vi "Main.vi"() -> ()   [LabVIEW 2020]
uses:
  <userlib>/_NEVSTOP/Communicable State Machine(CSM)/AdvanceAPI/CSM - Revert Arguments-Safe String.vi
  <userlib>/_NEVSTOP/Communicable State Machine(CSM)/_Support/Common/Trim Single line Text.vi
  <userlib>/_NEVSTOP/Communicable State Machine(CSM)/AdvanceAPI/CSM - Make String Arguments Safe.vi
  <userlib>/_NEVSTOP/Communicable State Machine(CSM)/AdvanceAPI/CSM - Break Down Multiple States String.vi
  <userlib>/_NEVSTOP/Communicable State Machine(CSM)/AdvanceAPI/CSM - Compact Multiple States.vi
  <userlib>/_NEVSTOP/Communicable State Machine(CSM)/AdvanceAPI/CSM - Keywords.vi
  <userlib>/_NEVSTOP/Communicable State Machine(CSM)/_Support/CSMQ/_CSMOFGV.vi
  <userlib>/_NEVSTOP/Communicable State Machine(CSM)/Communicable State Machine.lvlib
panel:
  out "State History":string
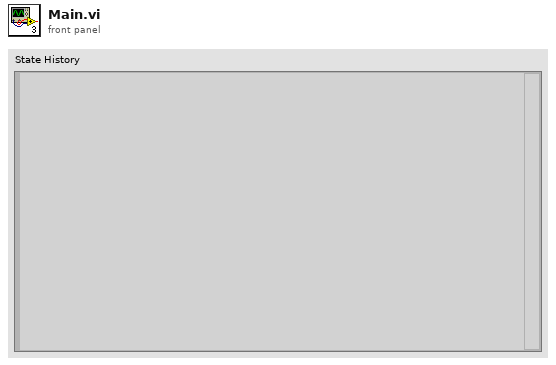
[diagram p1: front panel]
types:
  T1 = enum32{"Invalid", "Standard", "Closed", "Hidden", "Minimized", "Maximized"}
  T2 = enum32{"invalid app kind", "Development System", "Run Time System", "Student Edition", "Embedded LabVIEW", "Evaluation", "Custom"}
  T3 = typedef "Communicable State Machine.lvlib/_CSM_Response Source Message.ctl" = cluster{"‘State":string, "’Arguments":string, "’Error":errorcluster}
  T4 = cluster{"Current VI Reference":refnum<vi>, "Close Panel on Exit?":bool}
  T5 = cluster{"Core":cluster{"Current VI Reference":refnum<vi>, "Close Panel on Exit?":bool}, "Your Boolean data":bool, "Your string data":string}
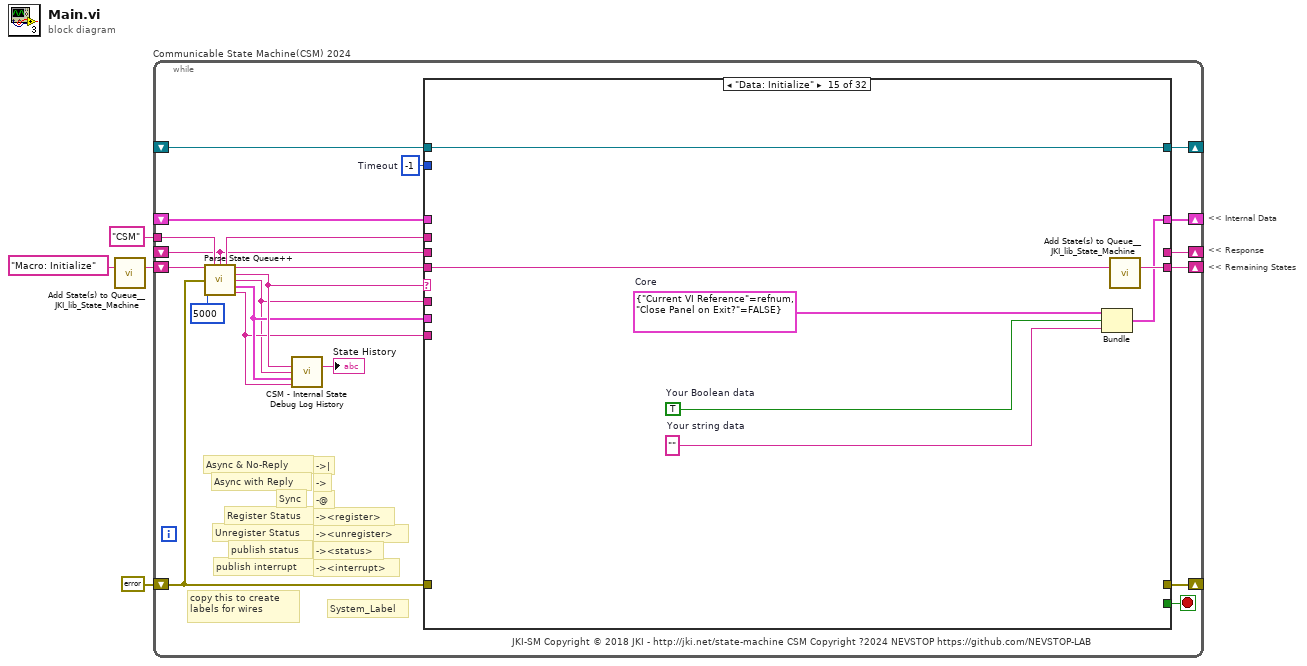
[diagram p0: block diagram]
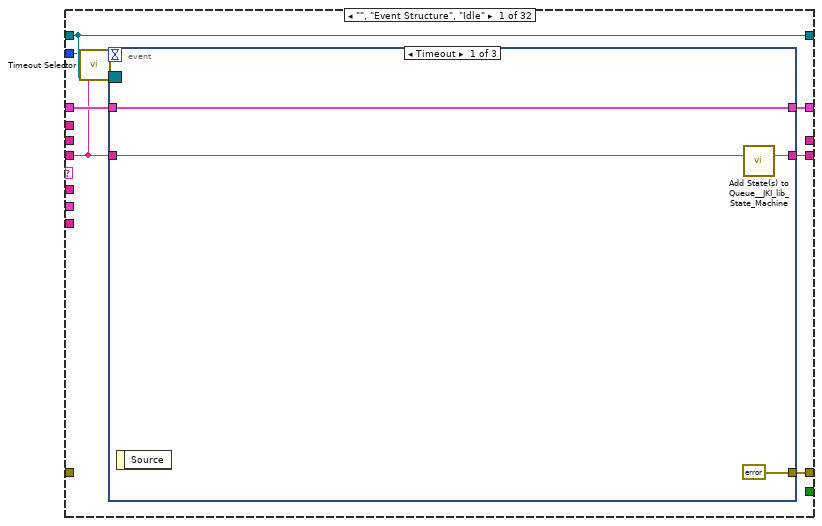
[diagram p2: hidden frame]
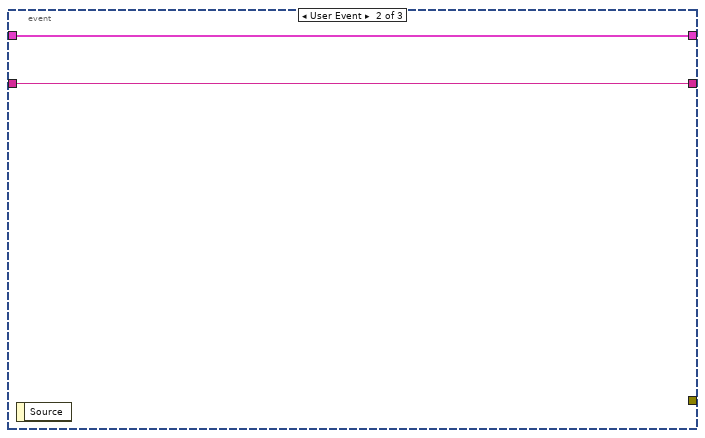
[diagram p3: hidden frame]
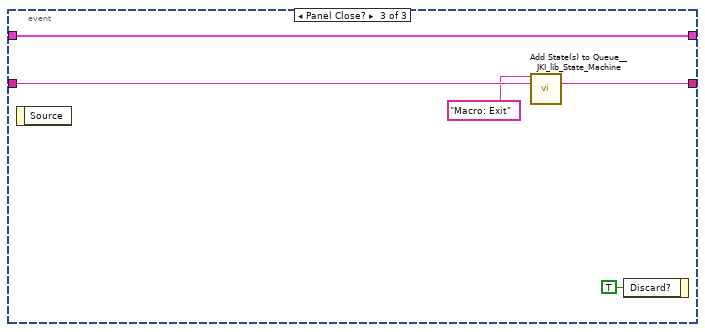
[diagram p4: hidden frame]
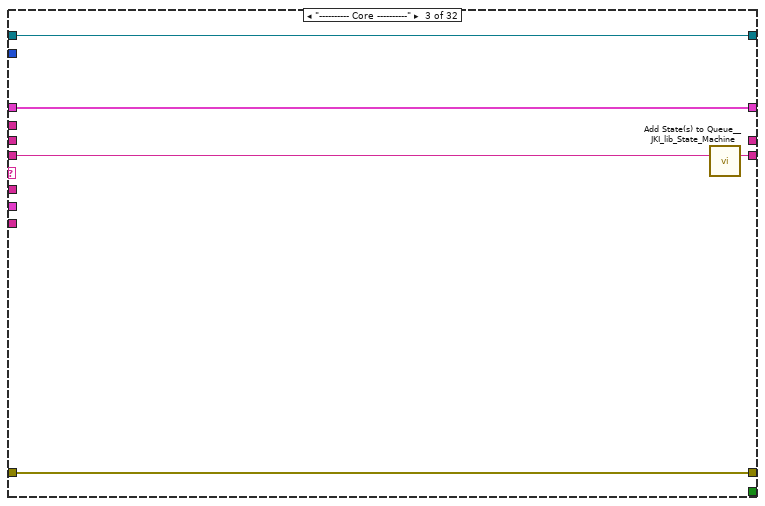
[diagram p6: hidden frame]
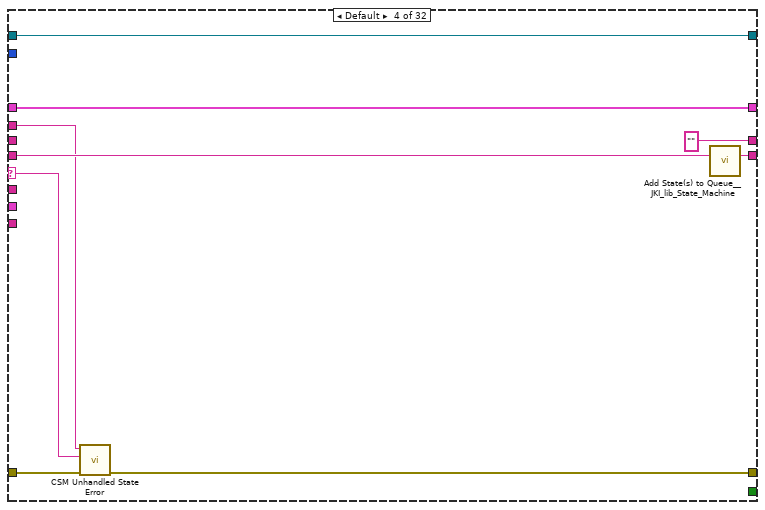
[diagram p7: hidden frame]
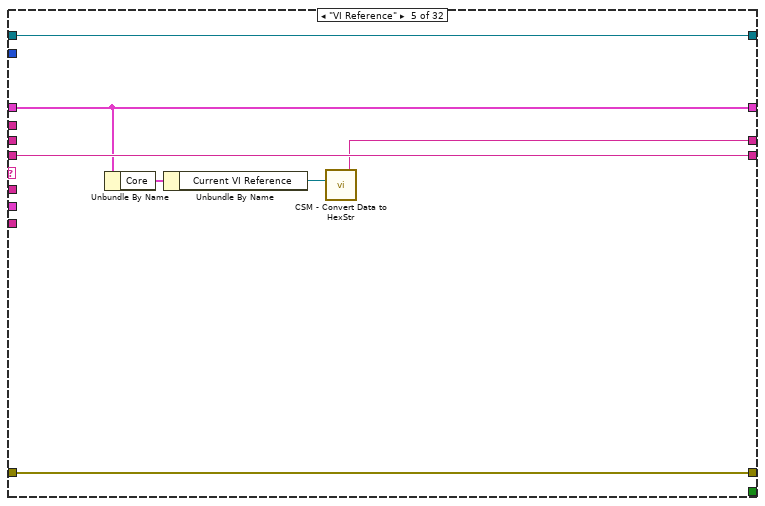
[diagram p8: hidden frame]
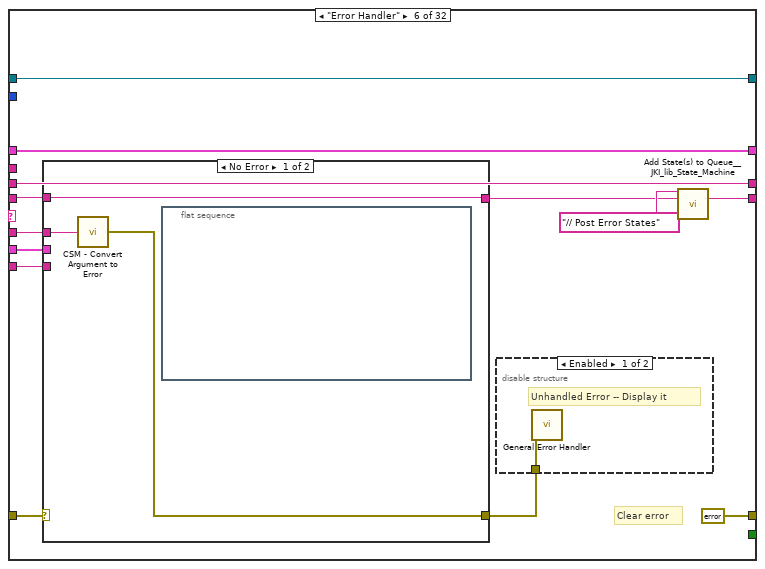
[diagram p9: hidden frame]
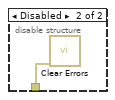
[diagram p10: hidden frame]
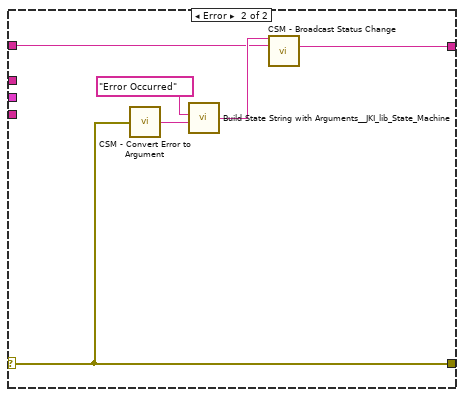
[diagram p11: hidden frame]
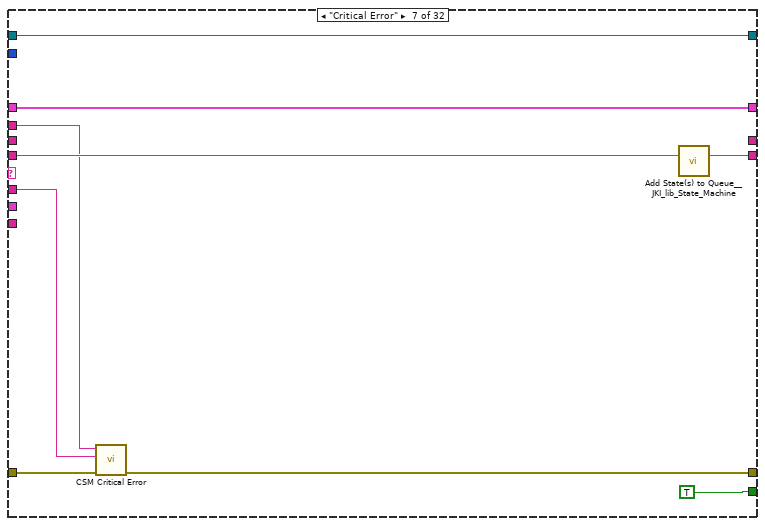
[diagram p12: hidden frame]
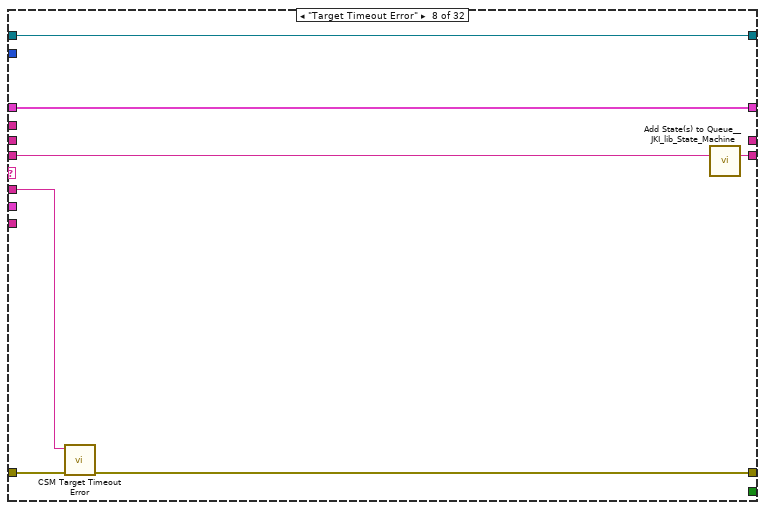
[diagram p13: hidden frame]
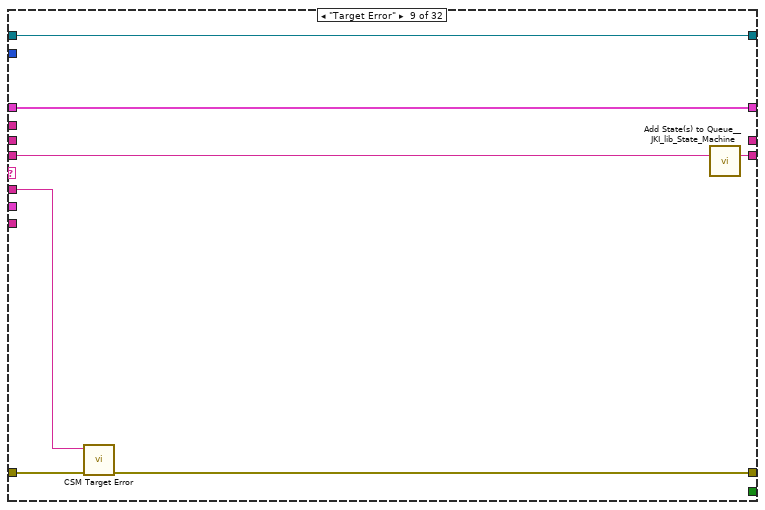
[diagram p14: hidden frame]
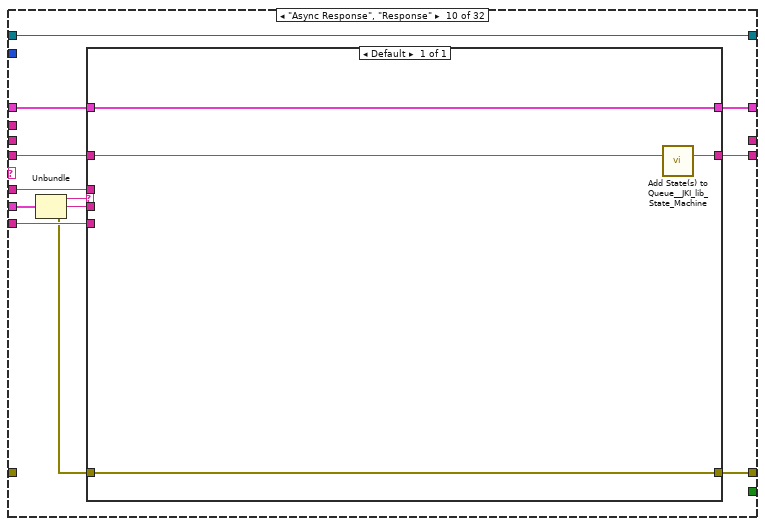
[diagram p15: hidden frame]
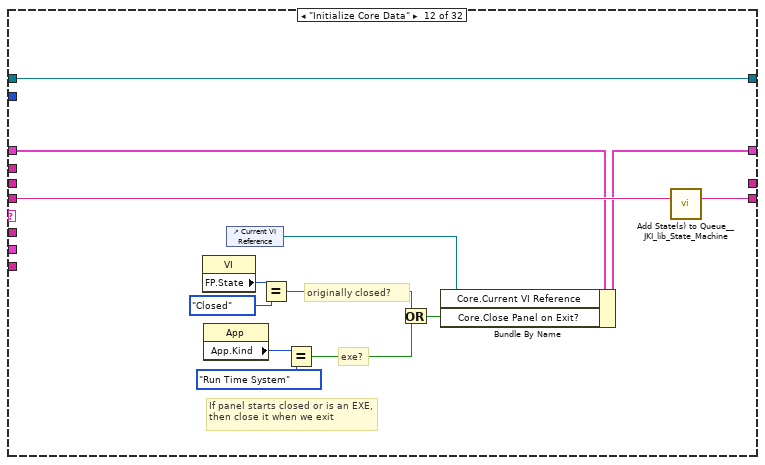
[diagram p17: hidden frame]
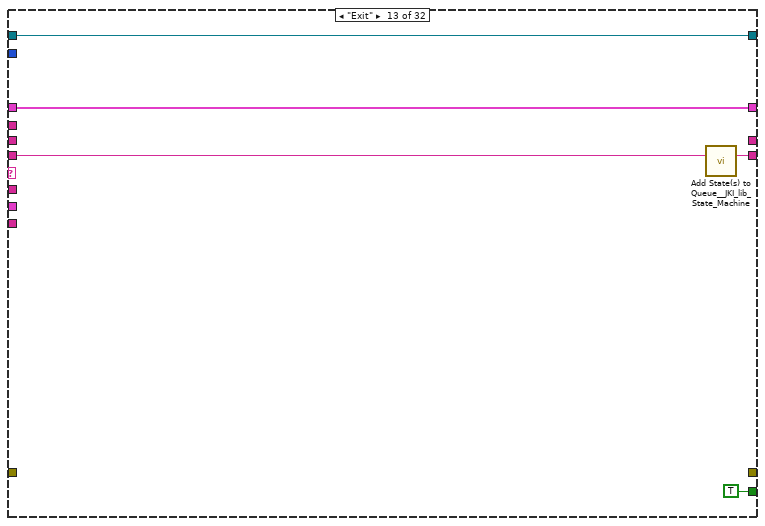
[diagram p18: hidden frame]
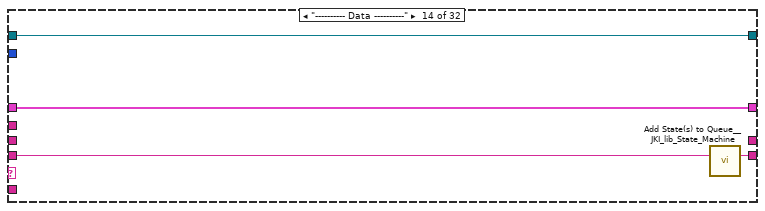
[diagram p19: hidden frame]
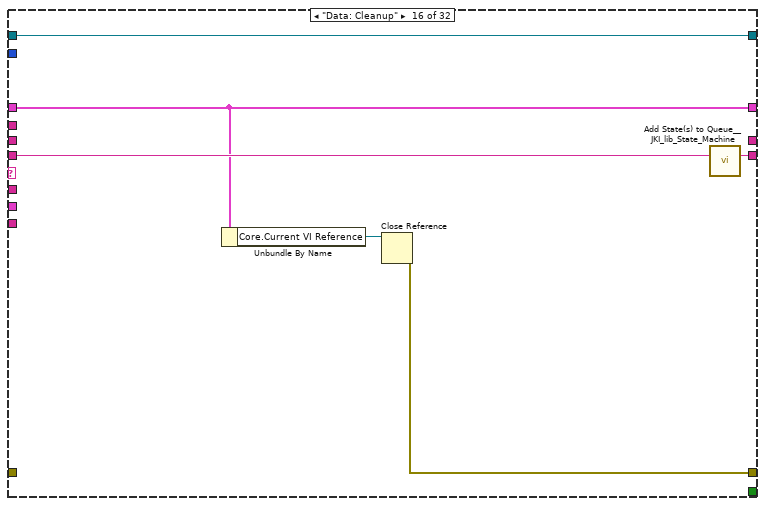
[diagram p20: hidden frame]
diagram:
  # "<< Internal Data"
  # "<< Response"
  # "<< Remaining States"
  n1 = call <vilib>:"Add State(s) to Queue__JKI_lib_State_Machine.vi"("State(s) in (\"\")"="Macro: Initialize" ("Init State(\"Macro: Initialize\")")) -> ("States Out"=w1:string)  [unwired: 14 in]
  n2 = while "Communicable State Machine(CSM) 2024" {
    shift-right: [w20] -> _
    shift-left: _ -> [w19]
    shift-right: [w23] -> _
    shift-left: errorcluster {"status"=FALSE, "code"=0, "source"=""} ("error out") -> [w17]
    shift-right: [w22] -> _
    shift-left: w1 -> [w24]
    tunnel: "CSM" ("Name(\"\" to use uuid)") -> [w12]
    shift-right: [w15] -> _
    shift-left: _ -> [w7]
    shift-right: [w14] -> _
    shift-left: _ -> [w13]
    stop <- w21 stop-if-true
    w18 = -1  # Timeout
    # "-><interrupt>"
    # "-><status>"
    # "-><unregister>"
    # "-><register>"
    # "-@"
    # "->"
    # "->|"
    # "publish interrupt"
    # "publish status"
    # "Unregister Status"
    # "Register Status"
    # "Sync"
    # "Async with Reply"
    # "Async & No-Reply"
    # "copy this to create labels for wires"
    # "System_Label"
    # "JKI-SM Copyright © 2018 JKI - http://jki.net/state-machine CSM Copyright ?2024 NEVSTOP https://github.com/NEVSTOP-LAB"
    n3 = call <userlib>:"Parse State Queue++.vi"("State Queue"=w24, "Name(\"\" to use uuid)"=w12, "Response Arguments"=w7, "Previous Error"=w17, "Response Timeout(5000ms)"=5000 ("Response Timeout(1000ms)")) -> ("Name Used"=w8:string, "Remaining States"=w25:string, "Current State"=w11:string, "Arguments"=w6:string, ">> Response Source Message >>"=w10:T3, ">> Source CSM >>"=w9:string)  [unwired: 5 in]
    n4 = call <userlib>:"CSM - Internal State Debug Log History.vi"("State"=w11, "Arguments (\"\")"=w6, ">> Response Source Message >>"=w10, "Source (\"\")"=w9) -> ("Debug Log"=→"State History":string)  [unwired: 11 in]
    n5 = case shown="\"Data: Initialize\"" w11 {
      selector: w11 -> [_ _ _ w55 _ _ _ _ _ _ _ _ _ _ _ _ _ _ _ _ _ _ _ _ _ _ _ _ _ _ _ _]
      tunnel: w25 -> [w26 w47 w52 w61 w67 w74 w100 w108 w115 w125 w134 w147 w152 w156 w163 w169 w173 w180 w184 w188 w192 w198 w209 w273 w278 w289 w292 w296 w299 w303 w307 w311]
      tunnel: w6 -> [_ _ _ _ _ w72 w96 w103 w111 w119 _ _ _ _ _ _ _ _ _ _ _ w194 w204 _ _ _ _ _ _ _ _ _]
      tunnel: w19 -> [w32 w46 w49 w59 w66 w80 w101 w106 w113 w123 w133 w141 w150 w154 _ w165 w171 w179 w183 w186 w190 w196 w206 w271 w276 w287 w291 w295 w298 w301 w305 w309]
      tunnel: [w31 _ w50 w53 w68 errorcluster {"status"=FALSE, "code"=0, "source"=""} ("error out") w93 w102 w109 w122 _ _ _ _ _ w166 _ w174 w182 _ _ w195 w207 _ _ _ _ _ _ _ _ _] -> w23
      tunnel: w17 -> [_ _ w50 w54 w68 w78 w94 w104 w110 _ _ _ _ _ _ _ _ _ _ _ _ _ _ _ _ _ _ _ _ _ _ _]
      tunnel: [w33 w47 w51 w60 w67 w76 w99 w107 w114 w126 w134 w146 w151 w155 w162 w168 w172 w180 w184 w187 w191 w197 w208 w272 w277 w288 w292 w296 w299 w302 w306 w310] -> w22
      tunnel: [_ _ _ _ _ _ TRUE _ _ _ _ _ TRUE _ _ _ _ _ _ _ _ _ _ _ _ _ _ _ _ _ _ _] -> w21
      tunnel: [w30 w46 w49 w59 w66 w80 w101 w106 w113 w124 w133 w145 w150 w154 w161 w165 w171 w179 w183 w186 w190 w196 w206 w271 w276 w287 w291 w295 w298 w301 w305 w309] -> w20
      tunnel: w18 -> [w28 _ _ _ _ _ _ _ _ _ _ _ _ _ _ _ _ _ _ _ _ _ _ _ _ _ _ _ _ _ _ _]
      tunnel: w9 -> [_ _ _ _ _ w71 _ _ _ w120 _ _ _ _ _ _ _ _ _ _ _ _ _ _ _ _ _ _ _ _ _ _]
      tunnel: w10 -> [_ _ _ _ _ w70 _ _ _ w121 _ _ _ _ _ _ _ _ _ _ _ _ _ _ _ _ _ _ _ _ _ _]
      tunnel: [_ _ _ "" w62 w69 _ _ _ _ _ _ _ _ _ _ _ _ _ _ _ _ _ _ _ _ _ "API1 Response" _ _ _ _] -> w15
      tunnel: [w29 w45 w48 w57 w65 w79 w97 w105 w112 w127 w132 w135 w148 w153 w157 w164 w170 w178 w181 w185 w189 w193 w203 w270 w274 w280 w290 w294 w297 w300 w304 w308] -> w14
      tunnel: w13 -> [w29 w45 w48 w57 w65 w79 w97 w105 w112 w127 w132 w135 w148 w153 w157 w164 w170 _ w181 w185 w189 w193 w203 w270 w274 w280 w290 w294 w297 w300 w304 w308]
      tunnel: w8 -> [_ _ _ w56 _ _ w95 _ _ _ _ _ _ _ _ _ _ w177 _ _ _ _ _ _ _ _ _ _ _ _ _ _]
      tunnel: w7 -> [_ _ _ _ _ w69 _ _ _ _ _ _ _ _ _ _ _ _ _ _ _ _ _ _ _ _ _ _ _ _ _ _]
      frame "", "Event Structure", "Idle" {
        n6 = call <userlib>:"Timeout Selector.vi"("Remaining States"=w26, "Timeout Expected"=w28) -> ("Timeout"=w27:i32)  [unwired: 5 in]
        n7 = event shown="[0] Timeout" {
          selector: w29 -> [_ _ _]
          dyn-events: _ -> [_ _ _]
          timeout: w27 -> [_ _ _]
          tunnel: w26 -> [w37 w38 w44]
          tunnel: [w36 w38 w43] -> w33
          tunnel: w32 -> [w35 w39 w42]
          tunnel: [errorcluster {"status"=FALSE, "code"=0, "source"=""} ("error out") _ _] -> w31
          tunnel: [w35 w39 w42] -> w30
          event Timeout {
            n8 = event-data() -> ()  [unwired: 1 in, 1 out]
            n9 = call <vilib>:"Add State(s) to Queue__JKI_lib_State_Machine.vi"("State(s) in (\"\")"=w37) -> ("States Out"=w36:string)  [unwired: 14 in]
          }
          event User Event {
            n10 = event-data() -> ()  [unwired: 1 in, 1 out]
          }
          event Panel Close? {
            n11 = event-data() -> ()  [unwired: 1 in, 1 out]
            n12 = call <vilib>:"Add State(s) to Queue__JKI_lib_State_Machine.vi"("State(s) in Front (\"\")"="Macro: Exit", "State(s) in (\"\")"=w44) -> ("States Out"=w43:string)  [unwired: 13 in]
            n13 = event-data("Discard?"=TRUE) -> ()  [unwired: 1 in, 1 out]
          }
        }
      }
      frame "CSM Documentation" {
      }
      frame "---------- Core ----------" {
        n14 = call <vilib>:"Add State(s) to Queue__JKI_lib_State_Machine.vi"("State(s) in (\"\")"=w52) -> ("States Out"=w51:string)  [unwired: 14 in]
      }
      frame Default {
        n15 = call <userlib>:"CSM Unhandled State Error.vi"("error in (no error)"=w54, "Current State"=w55, "CSM Name"=w56) -> ("error out"=w53:errorcluster)  [unwired: 8 in]
        n16 = call <vilib>:"Add State(s) to Queue__JKI_lib_State_Machine.vi"("State(s) in (\"\")"=w61) -> ("States Out"=w60:string)  [unwired: 14 in]
      }
      frame "VI Reference" {
        n17 = Unbundle By Name(w66) -> ("Core"=w64:T4)
        n18 = Unbundle By Name(w64) -> ("Current VI Reference"=w63:refnum<vi>)
        n19 = call <userlib>:"CSM - Convert Data to HexStr.vi"("Variant"=w63) -> ("HEX String (0-9,A-F)"=w62:string)  [unwired: 8 in]
      }
      frame "Error Handler" {
        # "Clear error"
        n20 = case shown="No Error" w78 {
          selector: w78 -> [_ w87]
          tunnel: [w85 w89] -> w75
          tunnel: w74 -> [w85 w88]
          tunnel: [w84 w87] -> w73
          tunnel: w72 -> [w86 _]
          tunnel: w71 -> [_ _]
          tunnel: w70 -> [_ _]
          frame No Error {
            n21 = call <userlib>:"CSM - Convert Argument to Error.vi"("Argument"=w86) -> ("error"=w84:errorcluster)  [unwired: 4 in]
            n22 = flat-sequence {
              frame #0 {
              }
            }
          }
          frame Error {
            n23 = call <userlib>:"CSM - Convert Error to Argument.vi"("error"=w87) -> ("Argument"=w91:string)  [unwired: 4 in]
            n24 = call <vilib>:"Build State String with Arguments__JKI_lib_State_Machine.vi"("Arguments (\"\")"=w91, "State"="Error Occurred" ("Status with Arguments")) -> ("State with Arguments"=w90:string)  [unwired: 4 in]
            n25 = call <userlib>:"CSM - Broadcast Status Change.vi"("Status with Arguments"=w90, "State Queue"=w88) -> ("Remaining States"=w89:string)  [unwired: 13 in]
          }
        }
        n26 = disable-structure shown="Enabled" {
          disable-tunnel: w73 -> [w82 w83]
          frame Enabled {
            # "Unhandled Error -- Display it"
            n27 = call <vilib>:"General Error Handler.vi"("error in (no error)"=w82) -> ()  [unwired: 10 in, 5 out]
          }
          frame Disabled {
            n28 = call <vilib>:"Clear Errors.vi"("error in (no error)"=w83) -> ()  [unwired: 5 in, 2 out]
          }
        }
        n29 = call <vilib>:"Add State(s) to Queue__JKI_lib_State_Machine.vi"("State(s) in Front (\"\")"="// Post Error States", "State(s) in (\"\")"=w75) -> ("States Out"=w76:string)  [unwired: 13 in]
      }
      frame "Critical Error" {
        n30 = call <userlib>:"CSM Critical Error.vi"("error in (no error)"=w94, "Arugments(as Reason)"=w96, "CSM Name"=w95) -> ("error out"=w93:errorcluster)  [unwired: 8 in]
        n31 = call <vilib>:"Add State(s) to Queue__JKI_lib_State_Machine.vi"("State(s) in (\"\")"=w100) -> ("States Out"=w99:string)  [unwired: 14 in]
      }
      frame "Target Timeout Error" {
        n32 = call <userlib>:"CSM Target Timeout Error.vi"("error in (no error)"=w104, "Arguments(as CSM Name)"=w103) -> ("error out"=w102:errorcluster)  [unwired: 9 in]
        n33 = call <vilib>:"Add State(s) to Queue__JKI_lib_State_Machine.vi"("State(s) in (\"\")"=w108) -> ("States Out"=w107:string)  [unwired: 14 in]
      }
      frame "Target Error" {
        n34 = call <userlib>:"CSM Target Error.vi"("error in (no error)"=w110, "Arguments(as CSM Name)"=w111) -> ("error out"=w109:errorcluster)  [unwired: 9 in]
        n35 = call <vilib>:"Add State(s) to Queue__JKI_lib_State_Machine.vi"("State(s) in (\"\")"=w115) -> ("States Out"=w114:string)  [unwired: 14 in]
      }
      frame "Async Response", "Response" {
        n36 = Unbundle(w121) -> ("‘State"=w118:string, "’Arguments"=w117:string, "’Error"=w116:errorcluster)
        n37 = case shown="Default" w118 {
          tunnel: [w128] -> w126
          tunnel: w125 -> [w129]
          tunnel: [w131] -> w124
          tunnel: w123 -> [w131]
          tunnel: [w130] -> w122
          tunnel: w116 -> [w130]
          tunnel: w120 -> [_]
          tunnel: w119 -> [_]
          tunnel: w117 -> [_]
          frame Default {
            n38 = call <vilib>:"Add State(s) to Queue__JKI_lib_State_Machine.vi"("State(s) in (\"\")"=w129) -> ("States Out"=w128:string)  [unwired: 14 in]
          }
        }
      }
      frame "Async Message Posted" {
      }
      frame "Initialize Core Data" {
        # "originally closed?"
        # "exe?"
        # "If panel starts closed or is an EXE, then close it when we exit"
        n39 = property class="VI"() -> ("FP.State"=w138:T1)  [unwired: 2 in, 2 out]
        n40 = property class="App"() -> ("App.Kind"=w144:T2)  [unwired: 2 in, 2 out]
        n41 = control-ref of="Current VI Reference"() -> (w139:refnum<vi>)
        n42 = Equal?(x=w138, y=T1."Closed" ("Front Panel Window:State")) -> (x = y?=w136:bool)
        n43 = Equal?(x=w144, y=T2."Run Time System" ("Application:Kind")) -> (x = y?=w142:bool)
        n44 = Or(x=w136, y=w142) -> (x .or. y?=w140:bool)
        n45 = Bundle By Name(cluster=w141, "Core.Current VI Reference"=w139, "Core.Close Panel on Exit?"=w140) -> (w145:T5)
        n46 = call <vilib>:"Add State(s) to Queue__JKI_lib_State_Machine.vi"("State(s) in (\"\")"=w147) -> ("States Out"=w146:string)  [unwired: 14 in]
      }
      frame "Exit" {
        n47 = call <vilib>:"Add State(s) to Queue__JKI_lib_State_Machine.vi"("State(s) in (\"\")"=w152) -> ("States Out"=w151:string)  [unwired: 14 in]
      }
      frame "---------- Data ----------" {
        n48 = call <vilib>:"Add State(s) to Queue__JKI_lib_State_Machine.vi"("State(s) in (\"\")"=w156) -> ("States Out"=w155:string)  [unwired: 14 in]
      }
      frame "Data: Initialize" {
        w158 = T4 {"Current VI Reference"=refnum, "Close Panel on Exit?"=FALSE}  # Core
        w160 = TRUE  # Your Boolean data
        w159 = ""  # Your string data
        n49 = Bundle("Core"=w158, "Your Boolean data"=w160, "Your string data"=w159) -> (w161:T5)  [unwired: 1 in]
        n50 = call <vilib>:"Add State(s) to Queue__JKI_lib_State_Machine.vi"("State(s) in (\"\")"=w163) -> ("States Out"=w162:string)  [unwired: 14 in]
      }
      frame "Data: Cleanup" {
        n51 = Unbundle By Name(w165) -> ("Core.Current VI Reference"=w167:refnum<vi>)
        n52 = Close Reference(reference=w167) -> (error out=w166:errorcluster)  [unwired: 1 in]
        n53 = call <vilib>:"Add State(s) to Queue__JKI_lib_State_Machine.vi"("State(s) in (\"\")"=w169) -> ("States Out"=w168:string)  [unwired: 14 in]
      }
      frame "---------- Events ----------" {
        n54 = call <vilib>:"Add State(s) to Queue__JKI_lib_State_Machine.vi"("State(s) in (\"\")"=w173) -> ("States Out"=w172:string)  [unwired: 14 in]
      }
      frame "Events: Register" {
        n55 = call <userlib>:"CSM - Get New State Notifier Event.vi"("Name(\"\" to use uuid) in"=w177) -> ("Error out"=w175:errorcluster, "New State Notifier Event"=w176:refnum<user-event>)  [unwired: 9 in]
        n56 = register-events(error in=w175, w176) -> (reference out=w178:refnum<event-registration>, error out=w174:errorcluster)  [unwired: 1 in]
      }
      frame "Events: Unregister" {
        n57 = Unregister For Events(event registration refnum=w181) -> (error out=w182:errorcluster)  [unwired: 1 in]
      }
      frame "---------- UI ----------" {
        n58 = call <vilib>:"Add State(s) to Queue__JKI_lib_State_Machine.vi"("State(s) in (\"\")"=w188) -> ("States Out"=w187:string)  [unwired: 14 in]
      }
      frame "UI: Initialize" {
        n59 = call <vilib>:"Add State(s) to Queue__JKI_lib_State_Machine.vi"("State(s) in (\"\")"=w192) -> ("States Out"=w191:string)  [unwired: 14 in]
      }
      frame "UI: Cursor Set" {
        # "Argument"
        n60 = disable-structure shown="Default" {
          disable-tunnel: [w200 _] -> w195
          disable-tunnel: w194 -> [w199 _]
          frame condition #0 (active) {
            n61 = case shown="\"Idle\", Default" w199 {
              tunnel: [w201 w202] -> w200
              frame "Idle", Default {
                n62 = call <vilib>:"Unset Busy.vi"() -> ("error out"=w201:errorcluster)  [unwired: 11 in]
              }
              frame "Busy" {
                n63 = call <vilib>:"Set Busy.vi"() -> ("error out"=w202:errorcluster)  [unwired: 10 in, 1 out]
              }
            }
          }
          frame condition #1 {
          }
        }
        n64 = call <vilib>:"Add State(s) to Queue__JKI_lib_State_Machine.vi"("State(s) in (\"\")"=w198) -> ("States Out"=w197:string)  [unwired: 14 in]
      }
      frame "UI: Front Panel State" {
        # "Argument"
        n65 = Unbundle By Name(w206) -> ("Core.Current VI Reference"=w205:refnum<vi>)
        n66 = case shown="\"Minimize\", \"Minimized\"" w204 {
          tunnel: [w216 w229 w240 w252 w264] -> w207
          tunnel: w205 -> [w215 w227 w239 w251 w263]
          frame "Open", "Standard", Default {
            w210 = T1."Standard" ("State")
            n67 = property class="VI"(reference=w215) -> (reference out=w213:refnum<vi>, error out=w214:errorcluster, "FP.State"=w212:T1)  [unwired: 1 in]
            n68 = Not Equal?(x=w212, y=w210) -> (x != y?=w211:bool)
            n69 = case shown="True" w211 {
              tunnel: [w220 w222] -> w216
              tunnel: w214 -> [w219 w222]
              tunnel: w213 -> [w218 _]
              tunnel: w210 -> [w217 _]
              frame True {
                n70 = invoke class="VI" method="FP.Open"(reference=w218, error in=w219, "Activate"=TRUE, "State"=w217) -> (error out=w220:errorcluster)  [unwired: 1 in, 4 out]
              }
              frame False {
              }
            }
          }
          frame "Close", "Closed" {
            n71 = property class="VI"(reference=w227) -> (reference out=w226:refnum<vi>, error out=w228:errorcluster, "FP.State"=w224:T1)  [unwired: 1 in]
            n72 = Not Equal?(x=w224, y=T1."Closed" ("Front Panel Window:State")) -> (x != y?=w223:bool)
            n73 = case shown="True" w223 {
              tunnel: [w230 w233] -> w229
              tunnel: w228 -> [w230 w232]
              tunnel: w226 -> [_ w231]
              frame False {
              }
              frame True {
                n74 = invoke class="VI" method="FP.Close"(reference=w231, error in=w232) -> (error out=w233:errorcluster)  [unwired: 1 in, 2 out]
              }
            }
          }
          frame "Hidden", "Hide" {
            w234 = T1."Hidden" ("State")
            n75 = property class="VI"(reference=w239) -> (reference out=w237:refnum<vi>, error out=w238:errorcluster, "FP.State"=w236:T1)  [unwired: 1 in]
            n76 = Not Equal?(x=w236, y=w234) -> (x != y?=w235:bool)
            n77 = case shown="True" w235 {
              tunnel: [w244 w245] -> w240
              tunnel: w238 -> [w243 w245]
              tunnel: w237 -> [w242 _]
              tunnel: w234 -> [w241 _]
              frame True {
                n78 = invoke class="VI" method="FP.Open"(reference=w242, error in=w243, "State"=w241) -> (error out=w244:errorcluster)  [unwired: 2 in, 4 out]
              }
              frame False {
              }
            }
          }
          frame "Minimize", "Minimized" {
            w246 = T1."Minimized" ("State")
            n79 = property class="VI"(reference=w251) -> (reference out=w249:refnum<vi>, error out=w250:errorcluster, "FP.State"=w248:T1)  [unwired: 1 in]
            n80 = Not Equal?(x=w248, y=w246) -> (x != y?=w247:bool)
            n81 = case shown="False" w247 {
              tunnel: [w256 w257] -> w252
              tunnel: w250 -> [w255 w257]
              tunnel: w249 -> [w254 _]
              tunnel: w246 -> [w253 _]
              frame True {
                n82 = invoke class="VI" method="FP.Open"(reference=w254, error in=w255, "State"=w253) -> (error out=w256:errorcluster)  [unwired: 2 in, 4 out]
              }
              frame False {
              }
            }
          }
          frame "Maximize", "Maximized" {
            w258 = T1."Maximized" ("State")
            n83 = property class="VI"(reference=w263) -> (reference out=w261:refnum<vi>, error out=w262:errorcluster, "FP.State"=w260:T1)  [unwired: 1 in]
            n84 = Not Equal?(x=w260, y=w258) -> (x != y?=w259:bool)
            n85 = case shown="True" w259 {
              tunnel: [w268 w269] -> w264
              tunnel: w262 -> [w267 w269]
              tunnel: w261 -> [w266 _]
              tunnel: w258 -> [w265 _]
              frame True {
                n86 = invoke class="VI" method="FP.Open"(reference=w266, error in=w267, "State"=w265) -> (error out=w268:errorcluster)  [unwired: 2 in, 4 out]
              }
              frame False {
              }
            }
          }
        }
        n87 = call <vilib>:"Add State(s) to Queue__JKI_lib_State_Machine.vi"("State(s) in (\"\")"=w209) -> ("States Out"=w208:string)  [unwired: 14 in]
      }
      frame "---------- Macro ----------" {
        n88 = call <vilib>:"Add State(s) to Queue__JKI_lib_State_Machine.vi"("State(s) in (\"\")"=w273) -> ("States Out"=w272:string)  [unwired: 14 in]
      }
      frame "Macro: Initialize" {
        w275 = "Data: Initialize\nInitialize Core Data\nEvents: Register\nUI: Initialize\nUI: Front Panel State >> Open"  # Data: Initialize Initialize Core Data Events: Register UI: Initialize UI: Front Panel State >> Open
        n89 = call <vilib>:"Add State(s) to Queue__JKI_lib_State_Machine.vi"("State(s) in Front (\"\")"=w275, "State(s) in (\"\")"=w278) -> ("States Out"=w277:string)  [unwired: 13 in]
      }
      frame "Macro: Exit" {
        n90 = Unbundle By Name(w287) -> ("Core.Close Panel on Exit?"=w286:bool)
        n91 = Select(t="UI: Front Panel State >> Close", s=w286, f="") -> (s? t:f=w283:string)
        n92 = call <vilib>:"Add State(s) to Queue__JKI_lib_State_Machine.vi"("State(s) in Front (\"\")"="//Exit Sub-Modules ", "State(s) in (\"\")"=w283, "State(s) at Back (\"\")"="Data: Cleanup\nEvents: Unregister\nExit") -> ("States Out"=w281:string)  [unwired: 12 in]
        n93 = call <vilib>:"Add State(s) to Queue__JKI_lib_State_Machine.vi"("State(s) in Front (\"\")"=w281, "State(s) in (\"\")"=w289) -> ("States Out"=w288:string)  [unwired: 13 in]
      }
      frame "---------- API ----------" {
      }
      frame "API: API1" {
      }
      frame "API: API2" {
      }
      frame "---------- Action ----------" {
        n94 = call <vilib>:"Add State(s) to Queue__JKI_lib_State_Machine.vi"("State(s) in (\"\")"=w303) -> ("States Out"=w302:string)  [unwired: 14 in]
      }
      frame "Action: action1" {
        n95 = call <vilib>:"Add State(s) to Queue__JKI_lib_State_Machine.vi"("State(s) in (\"\")"=w307) -> ("States Out"=w306:string)  [unwired: 14 in]
      }
      frame "Action: action2" {
        n96 = call <vilib>:"Add State(s) to Queue__JKI_lib_State_Machine.vi"("State(s) in (\"\")"=w311) -> ("States Out"=w310:string)  [unwired: 14 in]
      }
    }
  }
